vi "HexArray to HexString.vi"(0 "Hex Array In":u8[](array[numeric]) format="%.0x") -> (4 "Hex String Out":string)   [LabVIEW 2016]
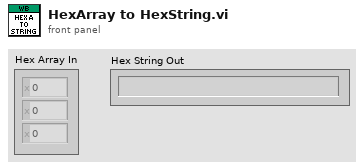
[diagram p1: front panel]
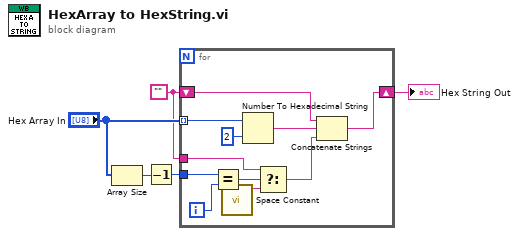
[diagram p0: block diagram]
diagram:
  w2 = ""
  n1 = Array Size(array="Hex Array In") -> (size(s)=w4:i32)
  n2 = Decrement(x=w4) -> (x-1=w3:i32)
  n3 = for {
    tunnel: "Hex Array In" -> [w16] mode=indexing
    shift-right: [w7] -> w1
    shift-left: w2 -> [w13]
    tunnel: w3 -> [w11]
    tunnel: w2 -> [w9]
    i -> [w12]
    n4 = Equal?(x=w11, y=w12) -> (x = y?=w6:bool)
    n5 = call <vilib>:"Space Constant.vi"() -> ("String"=w10:string)
    n6 = Number To Hexadecimal String(1:i16 2 ("width (-)"), 2:w16) -> (0:w14:string)
    n7 = Select(t=w9, s=w6, f=w10) -> (s? t:f=w8:string)
    n8 = Concatenate Strings(w13, w14, w8) -> (w7:string)
  }
  "Hex String Out" <- w1
